vi "CODMn电源命令.vi"(10 "通电/断电":bool, 11 "队列":refnum<queue>) -> (3 "队列输出":refnum<queue>)   [LabVIEW 2016, in "PLC.lvlib"]
uses:
  PLC.lvlib
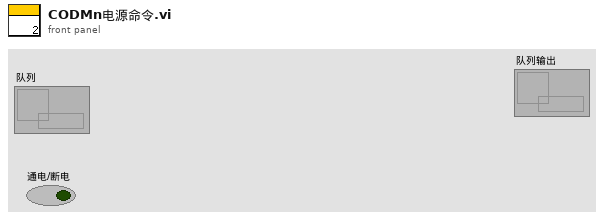
[diagram p1: front panel]
types:
  T1 = typedef "采配水类型.ctl" = enum16{"V1", "V2", "V3", "V4", "室内V1", "室内V2", "固定站V1", "固定站V2", "浮船V1", "浮船V2"}
  T2 = cluster{"命令":string, "data":cluster{"starting address":u16, "coil values":bool[]}}
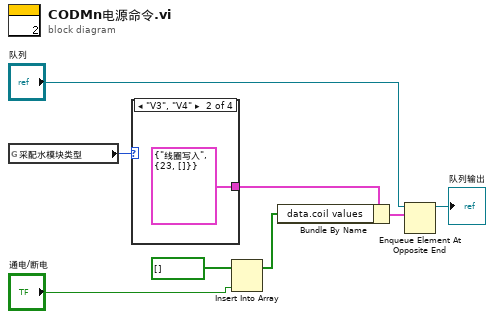
[diagram p0: block diagram]
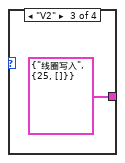
[diagram p3: hidden frame]
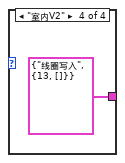
[diagram p4: hidden frame]
diagram:
  n1 = global read "系统设置全局变量.vi" "采配水模块类型"() -> (w1:T1)
  n2 = case shown="\"V3\", \"V4\"" w1 {
    tunnel: [_ T2 {"命令"="线圈写入", "data"={"starting address"=23, "coil values"=[]}} ("元素") T2 {"命令"="线圈写入", "data"={"starting address"=25, "coil values"=[]}} ("元素") T2 {"命令"="线圈写入", "data"={"starting address"=13, "coil values"=[]}} ("元素")] -> w8
    frame "V1", Default {
    }
    frame "V3", "V4" {
    }
    frame "V2" {
    }
    frame "室内V2" {
    }
  }
  n3 = Insert Into Array(array=bool[] [] ("data.coil values"), new element="通电/断电") -> (w3:bool[])  [unwired: 1 in]
  n4 = Bundle By Name(cluster=w8, "data.coil values"=w3) -> (w7:T2)
  n5 = Enqueue Element At Opposite End(queue="队列", element=w7) -> (queue out=→"队列输出":refnum<queue>)  [unwired: 2 in, 2 out]
